vi "Evaluate Unique ID.vi"(8 "error in (no error)":errorcluster, 11 "Unique ID":string) -> (0 "error out":errorcluster, 3 "Unique ID Out":string)   [LabVIEW 2019, in "Linked Lists.lvlib" / "Linked List.lvclass"]
uses:
  <vilib>/gpm_packages/@cs/linked-list/Source/Linked List/Linked List/Linked List.lvclass
  <vilib>/Utility/error.llb/Error Cluster From Error Code.vi
  <vilib>/ErrorRing/Error Ring.xnode
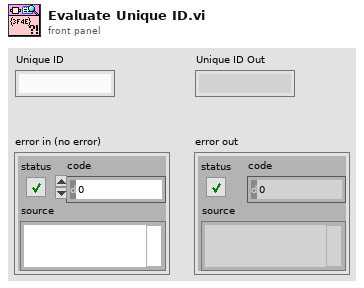
[diagram p1: front panel]
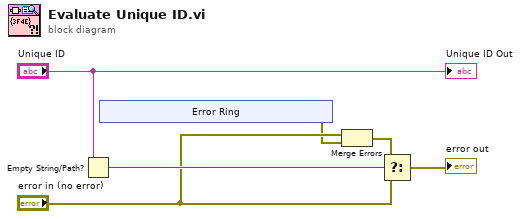
[diagram p0: block diagram]
diagram:
  n1 = Empty String/Path?(string/path="Unique ID") -> (empty?=w5:bool)
  n2 = xnode "Error Ring"() -> ("error out"=w3:errorcluster)
  n3 = Merge Errors("error in (no error)", w3) -> (w2:errorcluster)
  n4 = Select(t=w2, s=w5, f="error in (no error)") -> (s? t:f=→"error out":errorcluster)
  "Unique ID Out" <- "Unique ID"
